vi "АЛУ(пятиразрядное).vi"(3 "Func":T2, 4 "B":T3, 5 "A":T4) -> (0 "Type":bool, 1 "s1":bool, 2 "R":T1)   [LabVIEW 2013]
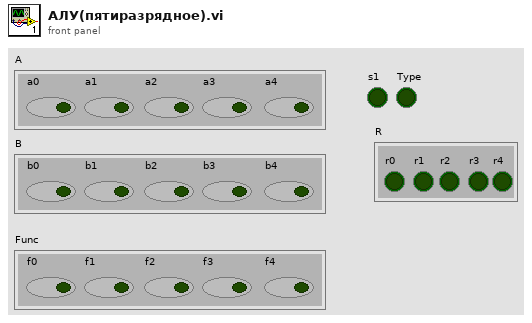
[diagram p1: front panel]
types:
  T1 = cluster{"r0":bool, "r1":bool, "r2":bool, "r3":bool, "r4":bool}
  T2 = cluster{"f0":bool, "f1":bool, "f2":bool, "f3":bool, "f4":bool}
  T3 = cluster{"b0":bool, "b1":bool, "b2":bool, "b3":bool, "b4":bool}
  T4 = cluster{"a0":bool, "a1":bool, "a2":bool, "a3":bool, "a4":bool}
  T5 = cluster{"r":bool, "r":bool, "r":bool, "r":bool, "r":bool}
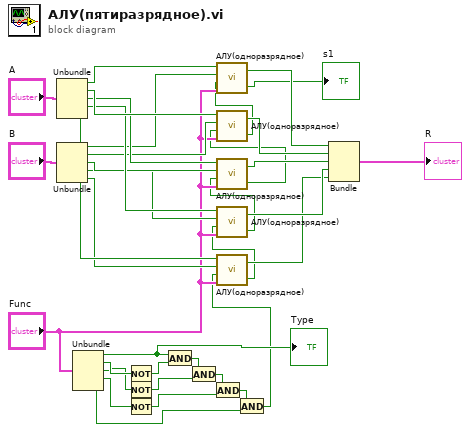
[diagram p0: block diagram]
diagram:
  n1 = Unbundle("A") -> ("a0"=w35:bool, "a1"=w34:bool, "a2"=w33:bool, "a3"=w32:bool, "a4"=w31:bool)
  n2 = Unbundle("B") -> ("b0"=w29:bool, "b1"=w28:bool, "b2"=w27:bool, "b3"=w26:bool, "b4"=w25:bool)
  n3 = Unbundle("Func") -> ("f0"=w7:bool, "f1"=w17:bool, "f2"=w16:bool, "f3"=w15:bool, "f4"=w8:bool)
  "Type" <- w7
  n4 = Not(x=w17) -> (.not. x?=w14:bool)
  n5 = Not(x=w16) -> (.not. x?=w10:bool)
  n6 = Not(x=w15) -> (.not. x?=w9:bool)
  n7 = And(x=w7, y=w14) -> (x .and. y?=w13:bool)
  n8 = And(x=w13, y=w10) -> (x .and. y?=w12:bool)
  n9 = And(x=w12, y=w9) -> (x .and. y?=w11:bool)
  n10 = And(x=w11, y=w8) -> (x .and. y?=w1:bool)
  n11 = call "АЛУ(одноразрядное).vi"("c"="Func", "c-1"=w1, "b"=w25, "a"=w31) -> ("s1"=w5:bool, "r"=w19:bool)
  n12 = call "АЛУ(одноразрядное).vi"("c"="Func", "c-1"=w5, "b"=w26, "a"=w32) -> ("s1"=w4:bool, "r"=w20:bool)
  n13 = call "АЛУ(одноразрядное).vi"("c"="Func", "c-1"=w4, "b"=w27, "a"=w33) -> ("s1"=w3:bool, "r"=w21:bool)
  n14 = call "АЛУ(одноразрядное).vi"("c"="Func", "c-1"=w3, "b"=w28, "a"=w34) -> ("s1"=w2:bool, "r"=w22:bool)
  n15 = call "АЛУ(одноразрядное).vi"("c"="Func", "c-1"=w2, "b"=w29, "a"=w35) -> ("s1"=→"s1":bool, "r"=w23:bool)
  n16 = Bundle("r"=w23, "r"=w22, "r"=w21, "r"=w20, "r"=w19) -> (→"R":T5)  [unwired: 1 in]
